vi "Configure Duty Cycle Correction.vi"(8 "error in (no error)":errorcluster, 10 "Duty Cycle Correction (1%)":dbl=1.0, 11 "VISA resource name":refnum<visa-resource-name>) -> (0 "error out":errorcluster, 3 "VISA resource name out":refnum<visa-resource-name>)   [LabVIEW 2018, in "Agilent U2000 Series.lvlib"]
doc: "Configures the duty cycle correction for the pulse power measurement feature of the U2000 Series power sensor.\n\nNote:\nThis VI is not applicable for Agilent U2021/2XA."
uses:
  Agilent U2000 Series.lvlib
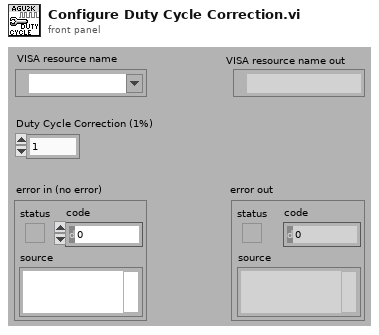
[diagram p1: front panel]
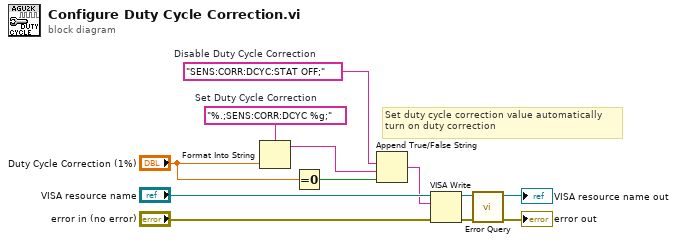
[diagram p0: block diagram]
diagram:
  w6 = "SENS:CORR:DCYC:STAT OFF;"  # Disable Duty Cycle Correction
  w10 = "%.;SENS:CORR:DCYC %g;"  # Set Duty Cycle Correction
  # "Set duty cycle correction value automatically\nturn on duty correction"
  n1 = Format Into String(format string=w10, "Duty Cycle Correction (1%)") -> (resulting string=w9:string)  [unwired: 2 in, 1 out]
  n2 = Equal To 0?(x="Duty Cycle Correction (1%)") -> (x = 0?=w8:bool)
  n3 = Append True/False String(1:w8, 2:w9, 3:w6) -> (0:w7:string)  [unwired: 1 out]
  n4 = VISA Write(VISA resource name="VISA resource name", write buffer=w7, error in (no error)="error in (no error)") -> (VISA resource name out=w3:refnum<visa-resource-name>, error out=w4:errorcluster)  [unwired: 1 out]
  n5 = call "Error Query.vi"("error in (no error)"=w4, "VISA resource name"=w3) -> ("error out"=→"error out":errorcluster, "VISA resource name out"=→"VISA resource name out":refnum<visa-resource-name>)  [unwired: 8 out]
